vi "Keithley 24XX Perform Statistical Operation.vi"() -> ()   [LabVIEW 2010]
doc: "Takes multiple points and performs a statistical operation on the data."
uses:
  <instrlib>/Keithley 24XX/Public/Data/Read (Statistical).vi
  <instrlib>/Keithley 24XX/Keithley 24XX.lvlib
panel:
  in  "Source Mode  (0: Voltage)":u16(ring) items=["Voltage", "Current"]
  out "Resistance Statistic":dbl
  out "Current Statistic":dbl
  out "Voltage Statistic":dbl
  in  "Statistical Operation (0: Mean)":u16(ring) items=["Mean", "Standard Deviation", "Maximum", "Minimum", "Peak to Peak"]
  in  "Output Level (0)":dbl
  in  "Compliance  Level (0.1)":dbl=0.1
  in  "Timeout (10000 ms)":i32=10000 format="%#.6g"
  in  "Sample Count (10)":i32=10
  in  "Serial Configuration":T1={"Baud Rate"=9600, "Parity"=0, "Data Bits"=8, "Stop Bits"=10, "Flow Control"=0} {"Flow Control" items=["None", "XON/XOFF", "RTS/CTS", "XON/XOFF & RTS/CTS", "DTR/DSR", "XON/XOFF & DTR/DSR"]; "Stop Bits" items=["1.0"=10, "1.5"=15, "2.0"=20]; "Data Bits" items=["7"=7, "8"=8]; "Parity" items=["None", "Odd", "Even", "Mark", "Space"]; "Baud Rate" items=["300"=300, "600"=600, "1200"=1200, "2400"=2400, "4800"=4800, "9600"=9600, "19200"=19200]}
  in  "VISA resource name":refnum<visa-resource-name>
  # "(c) 2006 - 2011 National Instruments.  ALL RIGHTS RESERVED."
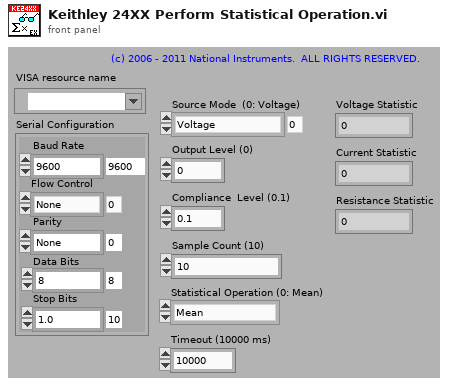
[diagram p1: front panel]
types:
  T1 = cluster{"Baud Rate":u32, "Parity":u16, "Data Bits":u16, "Stop Bits":u16, "Flow Control":u16}
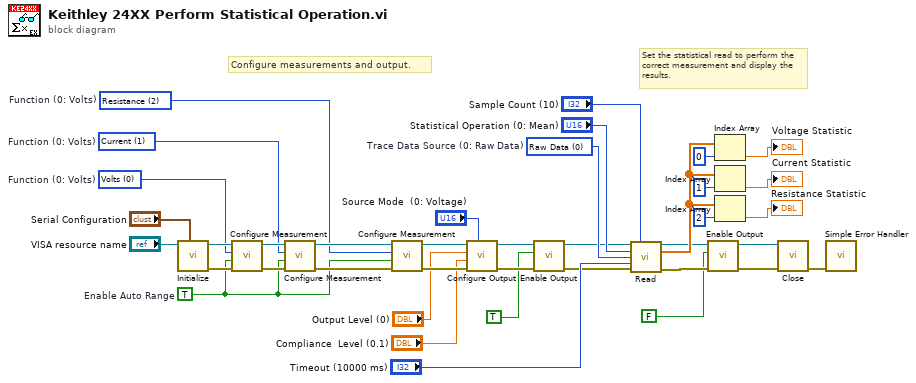
[diagram p0: block diagram]
diagram:
  w21 = u16 0 items=["Raw Data", "Math Data", "Limit Data"]  # Trace Data Source (0: Raw Data)
  w27 = u16 2 items=["Volts", "Current", "Resistance"]  # Function (0: Volts)
  w28 = u16 1 items=["Volts", "Current", "Resistance"]  # Function (0: Volts)
  w29 = u16 0 items=["Volts", "Current", "Resistance"]  # Function (0: Volts)
  w30 = TRUE  # Enable Auto Range
  # "Set the statistical read to perform the correct measurement and display the results."
  # "Configure measurements and output."
  n1 = call <instrlib>:"Initialize.vi"("Serial Configuration"="Serial Configuration", "VISA resource name"="VISA resource name") -> ("error out"=w36:errorcluster, "VISA resource name out"=w37:refnum<visa-resource-name>)  [unwired: 8 in]
  n2 = call <instrlib>:"Configure Measurement.vi"("error in (no error)"=w36, "Enable Auto Range (T:Enable)"=w30, "Function (0: Volts)"=w29, "VISA resource name"=w37) -> ("error out"=w34:errorcluster, "VISA resource name out"=w33:refnum<visa-resource-name>)  [unwired: 6 in]
  n3 = call <instrlib>:"Configure Measurement.vi"("error in (no error)"=w34, "Enable Auto Range (T:Enable)"=w30, "Function (0: Volts)"=w28, "VISA resource name"=w33) -> ("error out"=w31:errorcluster, "VISA resource name out"=w32:refnum<visa-resource-name>)  [unwired: 6 in]
  n4 = call <instrlib>:"Configure Measurement.vi"("error in (no error)"=w31, "Enable Auto Range (T:Enable)"=w30, "Function (0: Volts)"=w27, "VISA resource name"=w32) -> ("error out"=w24:errorcluster, "VISA resource name out"=w25:refnum<visa-resource-name>)  [unwired: 6 in]
  n5 = call <instrlib>:"Configure Output.vi"("Source Mode  (0: Voltage)"="Source Mode  (0: Voltage)", "error in (no error)"=w24, "Compliance  Level (0.1)"="Compliance  Level (0.1)", "Output Level (0)"="Output Level (0)", "VISA resource name"=w25) -> ("error out"=w10:errorcluster, "VISA resource name out"=w11:refnum<visa-resource-name>)  [unwired: 5 in]
  n6 = call <instrlib>:"Enable Output.vi"("error in (no error)"=w10, "Enable Output (T: Enable)"=TRUE, "VISA resource name"=w11) -> ("error out"=w9:errorcluster, "VISA resource name out"=w8:refnum<visa-resource-name>)  [unwired: 7 in]
  n7 = call-poly <instrlib>:"Read.vi"("VISA resource name"=w8, "Sample Count (2)"="Sample Count (10)", "Statistical Operation (0: Mean)"="Statistical Operation (0: Mean)", "Trace Data Source (0: Raw Data)"=w21, "Timeout (10000 ms)"="Timeout (10000 ms)", "error in (no error)"=w9) -> ("VISA resource name out"=w4:refnum<visa-resource-name>, "Statistical Operation Results"=w20:dbl[], "error out"=w5:errorcluster)  [unwired: 7 in]
  n8 = call <instrlib>:"Enable Output.vi"("error in (no error)"=w5, "Enable Output (T: Enable)"=FALSE, "VISA resource name"=w4) -> ("error out"=w7:errorcluster, "VISA resource name out"=w6:refnum<visa-resource-name>)  [unwired: 7 in]
  n9 = Index Array(array=w20, index=0) -> (element=→"Voltage Statistic":dbl)
  n10 = Index Array(array=w20, index=1) -> (element=→"Current Statistic":dbl)
  n11 = Index Array(array=w20, index=2) -> (element=→"Resistance Statistic":dbl)
  n12 = call <instrlib>:"Close.vi"("error in (no error)"=w7, "VISA resource name"=w6) -> ("error out"=w39:errorcluster)  [unwired: 9 in]
  n13 = call <vilib>:"Simple Error Handler.vi"("error in (no error)"=w39) -> ()  [unwired: 4 in, 5 out]
